vi "SecurityAcess RequestSeed.vi"(5 "LogSuspend":bool, 8 "error in":errorcluster, 11 "UdsHandleIn":T1={"LogPath"=path "", "LogEnabled"=FALSE, "isOpen"=FALSE, "LogContent"="", "Adapter"="CAN0", "MCanHandle"={"MCanAdapter"=refnum}, "TransmittId"=0, "ReceiveId"=0}) -> (0 "error out":errorcluster, 2 "Seed":string, 3 "UdsHandleOut":T1={"LogPath"=path "", "LogEnabled"=FALSE, "isOpen"=FALSE, "LogContent"="", "Adapter"="CAN0", "MCanHandle"={"MCanAdapter"=refnum}, "TransmittId"=0, "ReceiveId"=0})   [LabVIEW 2011, in "Konvolucio MUDS150628.lvlib"]
uses:
  <instrlib>/Konvolucio MUDS150628/Konvolucio MUDS150628.lvlib
  <instrlib>/Konvolucio MUDS150628/Types/UdsHandleType.ctl
  <instrlib>/Konvolucio MCAN120803/Types/MCanHandleType.ctl
  C:/Program Files/National Instruments/LabVIEW 2011/instr.lib/Konvolucio MCAN120803/Private/Konvolucio.MCAN120803.dll
  Konvolucio MCAN120803/Private/Konvolucio.MCAN120803.dll
  <instrlib>/Konvolucio MCAN120803/Konvolucio MCAN120803.lvlib
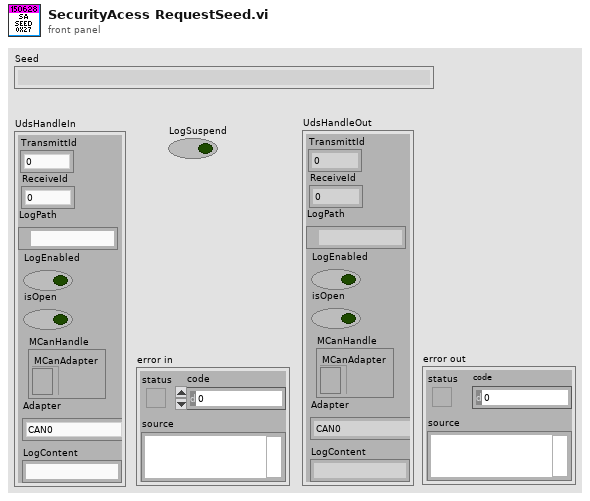
[diagram p1: front panel]
types:
  T1 = typedef "Konvolucio MUDS150628.lvlib/UdsHandleType.ctl" = cluster{"LogPath":path, "LogEnabled":bool, "isOpen":bool, "LogContent":string, "Adapter":string, "MCanHandle":T2, "TransmittId":u32, "ReceiveId":u32}
  T2 = typedef "Konvolucio MCAN120803.lvlib/MCanHandleType.ctl" = cluster{"MCanAdapter":refnum<k24>}
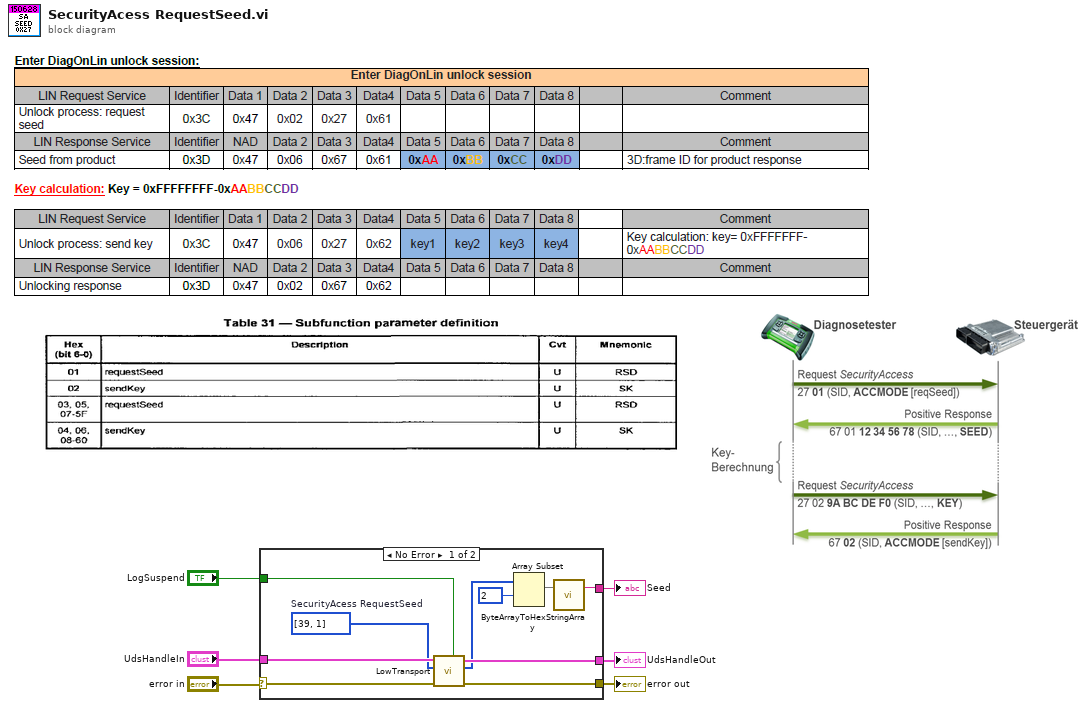
[diagram p0: block diagram]
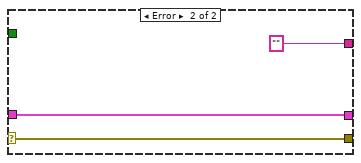
[diagram p2: hidden frame]
diagram:
  n1 = case shown="No Error" "error in" {
    selector: "error in" -> [w15 w19]
    tunnel: "UdsHandleIn" -> [w16 w18]
    tunnel: [w14 w19] -> w4
    tunnel: [w13 w18] -> w3
    tunnel: "LogSuspend" -> [w12 _]
    tunnel: [w8 "" ("HexStringArrayOut")] -> w1
    frame No Error {
      w11 = u8[] [39, 1]  # SecurityAcess RequestSeed
      n2 = call <instrlib>:"LowTransport.vi"("LogSuspend"=w12, "error in"=w15, "Request"=w11, "HandleIn"=w16) -> ("error out"=w14:errorcluster, "Response"=w10:u8[], "HandleOut"=w13:T1)  [unwired: 5 in]
      n3 = Array Subset(array=w10, index=2) -> (w7:u8[])  [unwired: 1 in]
      n4 = call <instrlib>:"ByteArrayToHexStringArray.vi"("ByteArrayIn"=w7) -> ("HexStringArrayOut"=w8:string)  [unwired: 2 in]
    }
    frame Error {
    }
  }
  "error out" <- w4
  "UdsHandleOut" <- w3
  "Seed" <- w1
